vi "L_vel_Control.vi"(8 "Loop time":dbl, 10 "Actual vel":i32, 11 "velocity":dbl) -> (3 "Current":i16)   [LabVIEW 2019]
uses:
  <vilib>/addons/control/pid/pid.llb/PID (DBL).vi
  <vilib>/addons/control/pid/NI_PID_pid.lvlib
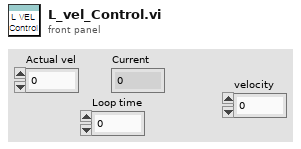
[diagram p1: front panel]
types:
  T1 = cluster{"proportional gain (Kc)":dbl, "integral time (Ti, min)":dbl, "derivative time (Td, min)":dbl}
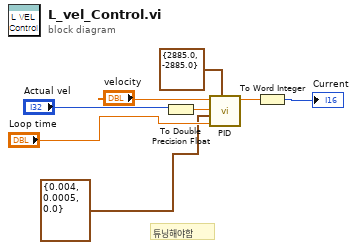
[diagram p0: block diagram]
diagram:
  # "튜닝해야함"
  n1 = To Double Precision Float(number="Actual vel") -> (double precision float=w3:dbl)
  n2 = call-poly <vilib>:"PID.vi"("output range"=cluster{"output high":dbl, "output low":dbl} {"output high"=2885.0, "output low"=-2885.0}, "dt (s)"="Loop time", "PID gains"=T1 {"proportional gain (Kc)"=0.004, "integral time (Ti, min)"=0.0005, "derivative time (Td, min)"=0.0}, "process variable"=w3, "setpoint"="velocity") -> ("output"=w7:dbl)  [unwired: 5 in, 1 out]
  n3 = To Word Integer(number=w7) -> (16bit integer=→"Current":i16)
